vi "save channels to interleaved tiff series.vi"(8 "frame number in":i32, 9 "last frame":bool, 11 "image data in":dbl[][](array[numeric])) -> ()   [LabVIEW 2012]
doc: "SciScan 1.2 160622"
uses:
  Custom Controls/file format type def.ctl
  GFG/GFGpathGet.vi
  GFG/GFGnumericGet.vi
  GFG/GFGstringGet.vi
  GFG/GFG library.lvlib
  Libtiff3/libtiff3.llb/libtiff3.lvlib
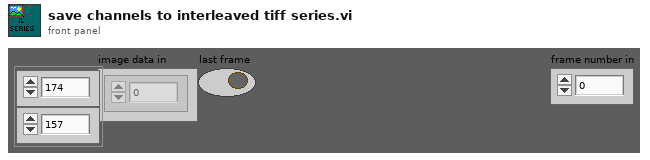
[diagram p1: front panel]
types:
  T1 = typedef "file format type def.ctl" = enum16{"16bit raw", "32bit raw", "16bit multi-tiff (interleave)", "16bit multi-tiff (separate)", "16bit multi-tiff (stacked)", "32bit multi-tiff (interleave)", "32bit multi-tiff (separate)", "32bit multi-tiff (stacked)", "16bit tiff series (interleave)", "16bit tiff series (separate)", "16bit tiff series (stacked)", "32bit tiff series (interleave)", "32bit tiff series (separate)", "32bit tiff series (stacked)"}
  T2 = cluster{"no..of.frames.to.acquire":dbl, "x.pixels":dbl, "y.pixels":dbl, "x.pixel.sz":dbl, "y.pixel.sz":dbl}
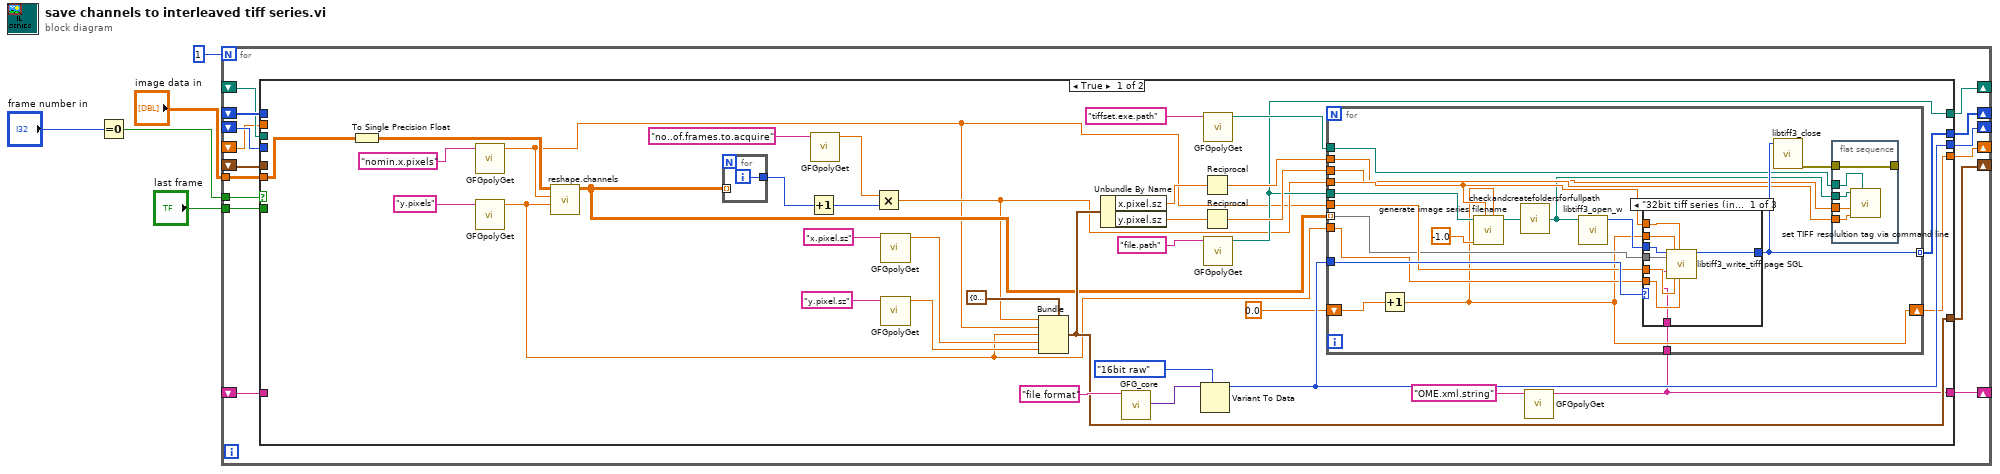
[diagram p0: block diagram]
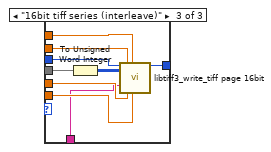
[diagram p3: hidden frame]
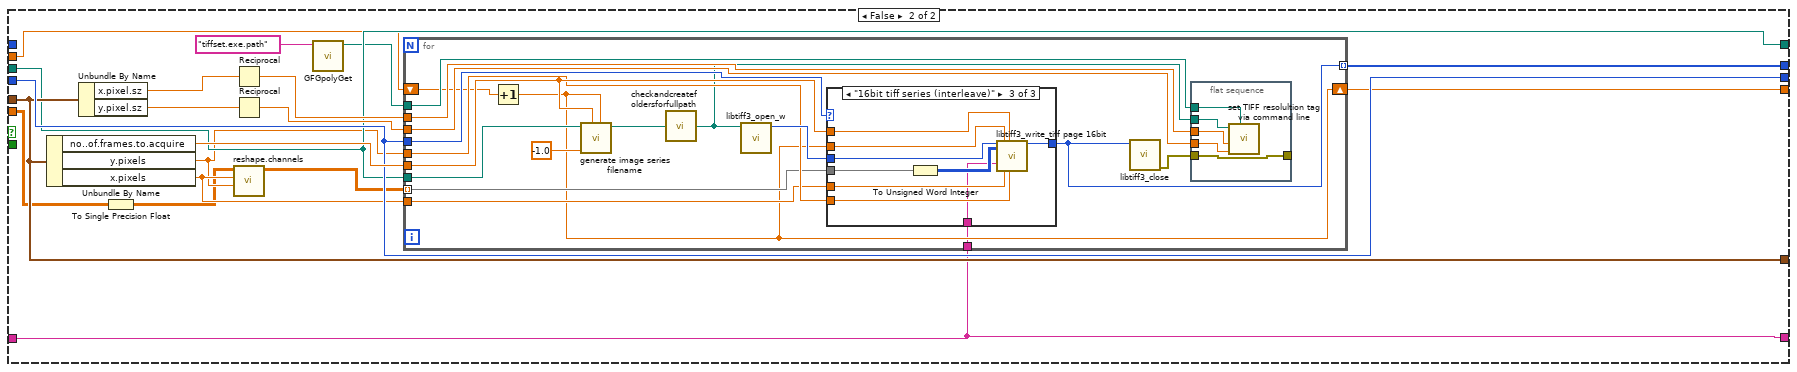
[diagram p4: hidden frame]
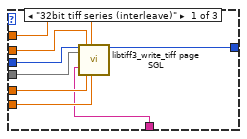
[diagram p5: hidden frame]
diagram:
  n1 = Equal To 0?(x="frame number in") -> (x = 0?=w4:bool)
  n2 = for {
    N: 1 -> [_]
    tunnel: w4 -> [w20]
    shift-right: [w19] -> _
    shift-left: _ -> [w18]
    tunnel: "image data in" -> [w17]
    shift-right: [w16] -> _
    shift-left: _ -> [w15]
    shift-right: [w14] -> _
    shift-left: _ -> [w13]
    shift-right: [w12] -> _
    shift-left: _ -> [w11]
    tunnel: "last frame" -> [w10]
    shift-right: [w9] -> _
    shift-left: _ -> [w8]
    shift-right: [w7] -> _
    shift-left: _ -> [w6]
    n3 = case shown="True" w20 {
      tunnel: w15 -> [_ w115]
      tunnel: [w42 w113] -> w19
      tunnel: w18 -> [_ _]
      tunnel: w17 -> [w32 w104]
      tunnel: [w43 w115] -> w16
      tunnel: [w41 w114] -> w14
      tunnel: w13 -> [_ w114]
      tunnel: [w34 w107] -> w12
      tunnel: w11 -> [_ w107]
      tunnel: w10 -> [_ _]
      tunnel: [w29 w99] -> w9
      tunnel: w8 -> [_ w100]
      tunnel: [w21 w98] -> w7
      tunnel: w6 -> [_ w98]
      frame True {
        n4 = To Single Precision Float(number=w32) -> (single precision float=w33:sgl[][])
        n5 = call-poly "GFGpolyGet.vi"("Variable Name in"="nomin.x.pixels" ("Tag in")) -> ("Numeric"=w23:dbl)  [unwired: 8 in, 2 out]
        n6 = call-poly "GFGpolyGet.vi"("Variable Name in"="y.pixels" ("Tag in")) -> ("Numeric"=w31:dbl)  [unwired: 8 in, 2 out]
        n7 = call "reshape.channels.vi"("y.pixels"=w31, "x.pixels"=w23, "element"=w33) -> ("Array"=w28:dbl[][][])  [unwired: 8 in]
        n8 = for {
          tunnel: w28 -> [_] mode=indexing
          tunnel: [w56] -> w26
          i -> [w56]
        }
        n9 = Increment(x=w26) -> (x+1=w25:i32)
        n10 = call-poly "GFGpolyGet.vi"("Variable Name in"="no..of.frames.to.acquire") -> ("Numeric"=w27:dbl)  [unwired: 8 in, 2 out]
        n11 = Multiply(x=w27, y=w25) -> (x*y=w24:dbl)
        n12 = call-poly "GFGpolyGet.vi"("Variable Name in"="x.pixel.sz" ("Tag in")) -> ("Numeric"=w46:dbl)  [unwired: 8 in, 2 out]
        n13 = call-poly "GFGpolyGet.vi"("Variable Name in"="y.pixel.sz" ("Tag in")) -> ("Numeric"=w45:dbl)  [unwired: 8 in, 2 out]
        n14 = Bundle(cluster=T2 {"no..of.frames.to.acquire"=0.0, "x.pixels"=0.0, "y.pixels"=0.0, "x.pixel.sz"=0.0, "y.pixel.sz"=0.0} ("output cluster"), "no..of.frames.to.acquire"=w24, "x.pixels"=w23, "y.pixels"=w31, "x.pixel.sz"=w46, "y.pixel.sz"=w45) -> (w41:T2)
        n15 = Unbundle By Name(w41) -> ("x.pixel.sz"=w37:dbl, "y.pixel.sz"=w38:dbl)
        n16 = call "GFG_core.vi"("Variable Name in"="file format") -> ("Variant Out"=w54:variant)  [unwired: 12 in, 6 out]
        n17 = Variant To Data(type=file_format_type_def."16bit raw" ("file format"), Variant=w54) -> (data=w43:T1)  [unwired: 1 in, 1 out]
        n18 = Reciprocal(x=w37) -> (1/x=w39:dbl)
        n19 = Reciprocal(x=w38) -> (1/x=w40:dbl)
        n20 = call-poly "GFGpolyGet.vi"("Variable Name in"="tiffset.exe.path") -> ("Path"=w35:path)  [unwired: 8 in, 2 out]
        n21 = call-poly "GFGpolyGet.vi"("Variable Name in"="file.path") -> ("Path"=w34:path)  [unwired: 8 in, 2 out]
        n22 = call-poly "GFGpolyGet.vi"("Variable Name in"="OME.xml.string" ("Tag in")) -> ("String"=w21:string)  [unwired: 9 in, 1 out]
        n23 = for {
          tunnel: w43 -> [w74]
          tunnel: w23 -> [w72]
          tunnel: w31 -> [w71]
          tunnel: w24 -> [w69]
          tunnel: [w68] -> w42 mode=indexing
          tunnel: w40 -> [w66]
          tunnel: w39 -> [w65]
          tunnel: w35 -> [w64]
          tunnel: w34 -> [w63]
          tunnel: w28 -> [w62] mode=indexing
          shift-right: [w58] -> w29
          shift-left: 0.0 -> [w60]
          tunnel: w21 -> [w57]
          n24 = Increment(x=w60) -> (x+1=w58:dbl)
          n25 = call "generate image series filename.vi"("frame number in"=w58, "no..of.frames.to.acquire"=w69, "channel"=-1.0, "Path IN"=w63) -> ("appended path"=w70:path)  [unwired: 7 in]
          n26 = call "checkandcreatefoldersforfullpath.vi"("Path IN"=w70) -> ("Path OUT"=w61:path)  [unwired: 4 in]
          n27 = call "libtiff3_open_w.vi"("Input path"=w61) -> ("handle"=w73:i32)  [unwired: 9 in, 1 out]
          n28 = case shown="\"32bit tiff series (interleave)\"" w74 {
            tunnel: w62 -> [w81 _ w94]
            tunnel: w73 -> [w84 w88 w95]
            tunnel: w58 -> [w85 _ w96]
            tunnel: w69 -> [w86 _ w97]
            tunnel: [w87 w88 w90] -> w68
            tunnel: w72 -> [w82 _ w92]
            tunnel: w71 -> [w83 _ w91]
            tunnel: w57 -> [w80 _ w89]
            frame "32bit tiff series (interleave)" {
              n29 = call "libtiff3_write_tiff page SGL.vi"("Handle"=w84, "Image Pixels (Float)"=w81, "Image Description"=w80, "page"=w85, "x.pixels"=w82, "totalpages"=w86, "y.pixels"=w83) -> ("Handle out"=w87:i32)  [unwired: 11 in, 1 out]
            }
            frame Default {
            }
            frame "16bit tiff series (interleave)" {
              n30 = To Unsigned Word Integer(number=w94) -> (unsigned 16bit integer=w93:u16[][])
              n31 = call "libtiff3_write_tiff page 16bit.vi"("Handle"=w95, "Image Pixels (U16)"=w93, "ImageDescription"=w89, "page"=w96, "x.pixels"=w92, "totalpages"=w97, "y.pixels"=w91) -> ("Handle out"=w90:i32)  [unwired: 11 in, 1 out]
            }
          }
          n32 = call "libtiff3_close.vi"("Handle"=w68) -> ("error out"=w67:errorcluster)  [unwired: 9 in]
          n33 = flat-sequence {
            tunnel: w67 -> [w77]
            tunnel: w65 -> [w79]
            tunnel: w66 -> [w78]
            tunnel: [w77] -> _
            tunnel: w64 -> [w76]
            tunnel: w61 -> [w75]
            frame #0 {
              n34 = call "set TIFF resolultion tag via command line.vi"("tiffset.exe file path"=w76, "y pixels per m"=w78, "x pixels per m"=w79, "TIFF file path"=w75) -> ()  [unwired: 8 in]
            }
          }
        }
      }
      frame False {
        n35 = Unbundle By Name(w114) -> ("no..of.frames.to.acquire"=w116:dbl, "y.pixels"=w105:dbl, "x.pixels"=w106:dbl)
        n36 = Unbundle By Name(w114) -> ("x.pixel.sz"=w109:dbl, "y.pixel.sz"=w110:dbl)
        n37 = To Single Precision Float(number=w104) -> (single precision float=w103:sgl[][])
        n38 = Reciprocal(x=w109) -> (1/x=w111:dbl)
        n39 = Reciprocal(x=w110) -> (1/x=w112:dbl)
        n40 = call "reshape.channels.vi"("y.pixels"=w105, "x.pixels"=w106, "element"=w103) -> ("Array"=w102:dbl[][][])  [unwired: 8 in]
        n41 = call-poly "GFGpolyGet.vi"("Variable Name in"="tiffset.exe.path") -> ("Path"=w101:path)  [unwired: 8 in, 2 out]
        n42 = for {
          tunnel: w116 -> [w132]
          tunnel: w115 -> [w131]
          tunnel: w105 -> [w130]
          tunnel: w106 -> [w129]
          tunnel: [w128] -> w113 mode=indexing
          tunnel: w112 -> [w126]
          tunnel: w111 -> [w125]
          tunnel: w107 -> [w124]
          tunnel: w102 -> [w123] mode=indexing
          tunnel: w101 -> [w122]
          shift-right: [w118] -> w99
          shift-left: w100 -> [w120]
          tunnel: w98 -> [w117]
          n43 = Increment(x=w120) -> (x+1=w118:dbl)
          n44 = call "generate image series filename.vi"("frame number in"=w118, "no..of.frames.to.acquire"=w132, "channel"=-1.0, "Path IN"=w124) -> ("appended path"=w133:path)  [unwired: 7 in]
          n45 = call "checkandcreatefoldersforfullpath.vi"("Path IN"=w133) -> ("Path OUT"=w121:path)  [unwired: 4 in]
          n46 = call "libtiff3_open_w.vi"("Input path"=w121) -> ("handle"=w134:i32)  [unwired: 9 in, 1 out]
          n47 = case shown="\"16bit tiff series (interleave)\"" w131 {
            tunnel: w123 -> [w141 _ w154]
            tunnel: w134 -> [w144 w148 w155]
            tunnel: w118 -> [w145 _ w156]
            tunnel: w132 -> [w146 _ w157]
            tunnel: [w147 w148 w150] -> w128
            tunnel: w129 -> [w142 _ w152]
            tunnel: w130 -> [w143 _ w151]
            tunnel: w117 -> [w140 _ w149]
            frame "32bit tiff series (interleave)" {
              n48 = call "libtiff3_write_tiff page SGL.vi"("Handle"=w144, "Image Pixels (Float)"=w141, "Image Description"=w140, "page"=w145, "x.pixels"=w142, "totalpages"=w146, "y.pixels"=w143) -> ("Handle out"=w147:i32)  [unwired: 11 in, 1 out]
            }
            frame Default {
            }
            frame "16bit tiff series (interleave)" {
              n49 = To Unsigned Word Integer(number=w154) -> (unsigned 16bit integer=w153:u16[][])
              n50 = call "libtiff3_write_tiff page 16bit.vi"("Handle"=w155, "Image Pixels (U16)"=w153, "ImageDescription"=w149, "page"=w156, "x.pixels"=w152, "totalpages"=w157, "y.pixels"=w151) -> ("Handle out"=w150:i32)  [unwired: 11 in, 1 out]
            }
          }
          n51 = call "libtiff3_close.vi"("Handle"=w128) -> ("error out"=w127:errorcluster)  [unwired: 9 in]
          n52 = flat-sequence {
            tunnel: w127 -> [w137]
            tunnel: w125 -> [w139]
            tunnel: w126 -> [w138]
            tunnel: [w137] -> _
            tunnel: w122 -> [w136]
            tunnel: w121 -> [w135]
            frame #0 {
              n53 = call "set TIFF resolultion tag via command line.vi"("tiffset.exe file path"=w136, "y pixels per m"=w138, "x pixels per m"=w139, "TIFF file path"=w135) -> ()  [unwired: 8 in]
            }
          }
        }
      }
    }
  }
